vi "Build Path.vi"(0 "Table path":string, 5 "Column path":string, 7 "Table name":string, 9 "Column name":string, 11 "Column units":string) -> (8 "PG path":string="llab_038:d001(TEST_TABLE--new_stuff(hippos))")   [LabVIEW 2013, in "Data.PGSQL.lvclass"]
uses:
  Data.PGSQL.lvclass
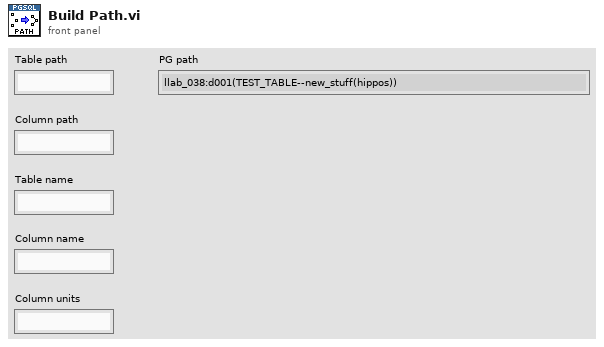
[diagram p1: front panel]
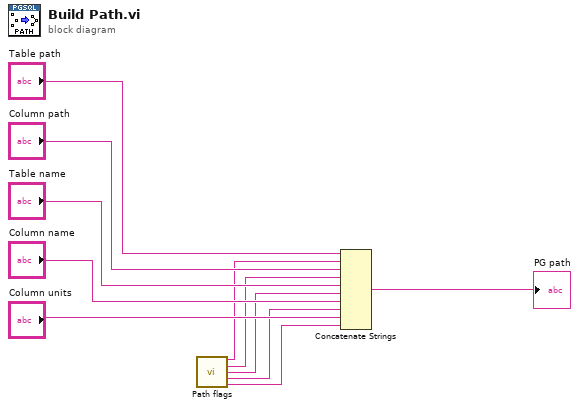
[diagram p0: block diagram]
diagram:
  n1 = call "Path flags.vi"() -> ("table_path()column_path"=w6:string, "column_path()table_name"=w5:string, "table_name()column_name"=w4:string, "column_name()units"=w3:string, "units()"=w2:string)  [unwired: 11 in]
  n2 = Concatenate Strings("Table path", w6, "Column path", w5, "Table name", w4, "Column name", w3, "Column units", w2) -> (→"PG path":string)
